vi "Simulation Resource Buffer.vi"(6 "IO Buffer Operation":T1, 8 "error in (no error)":errorcluster, 11 "Data in":variant) -> (0 "error out":errorcluster, 2 "Timed Out?":bool, 3 "Data out":variant)   [LabVIEW 2016]
uses:
  Typedefs/IO Buffer Operation.ctl
  Typedefs/IO Data Cluster.ctl
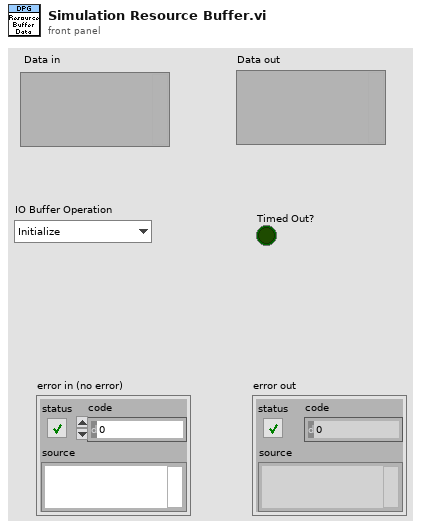
[diagram p1: front panel]
types:
  T1 = typedef "IO Buffer Operation.ctl" = enum16{"Initialize", "Write IO Data_Rd", "Read IO Data_Rd", "Write IO Data_Wr", "Read IO Data_Wr", "Write  IO Data_Dir", "Read  IO Data_Dir", "Write Host to Target FIFO", "Read Host to Target FIFO", "Write Target to Host FIFO", "Read Target to Host FIFO", "Write Monitor Enable?", "Read Monitor Enable?", "Close"}
  T2 = typedef "IO Data Cluster.ctl" = cluster{"Host to Target FIFO":refnum<queue>, "Target to Host FIFO":refnum<queue>, "Monitor Enable?":bool, "IO Data_Wr":refnum<queue>, "IO Data_Rd":refnum<queue>, "IO Data_Dir":u32}
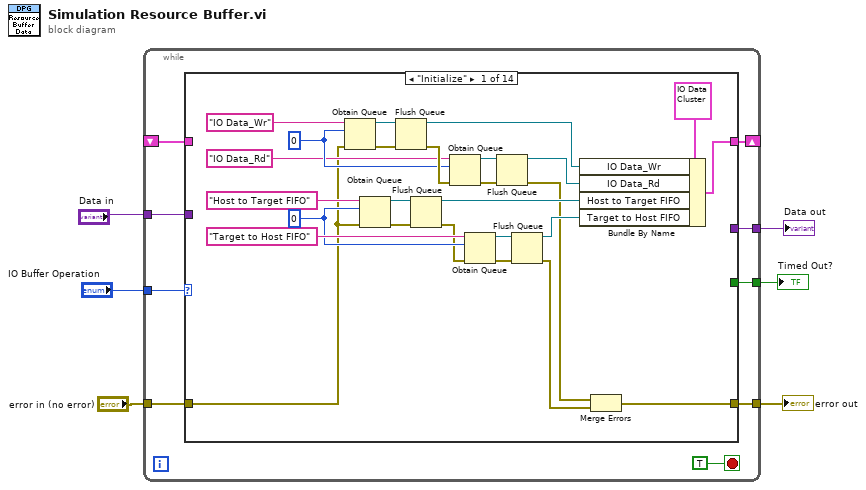
[diagram p0: block diagram]
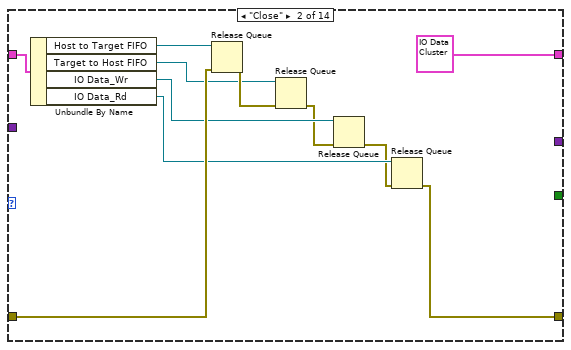
[diagram p2: hidden frame]
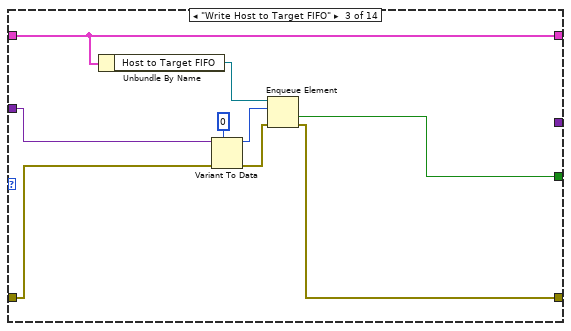
[diagram p3: hidden frame]
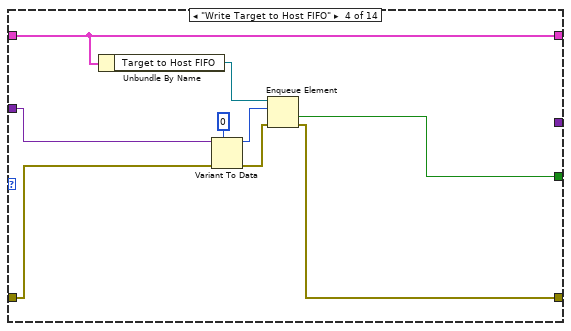
[diagram p4: hidden frame]
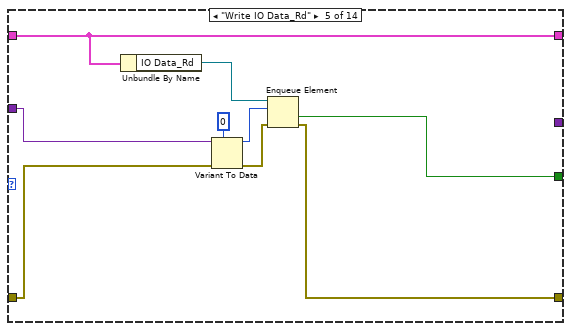
[diagram p5: hidden frame]
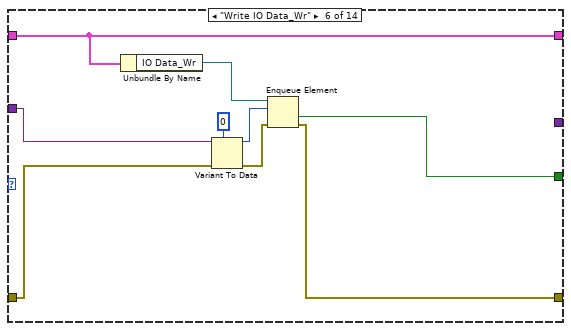
[diagram p6: hidden frame]
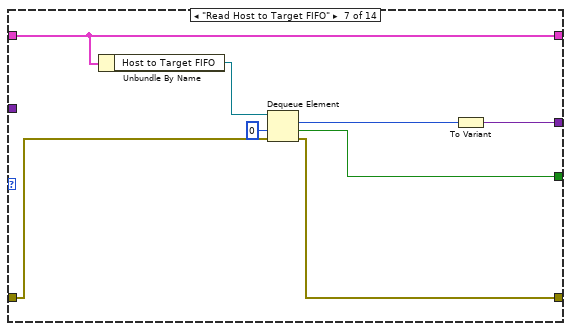
[diagram p7: hidden frame]
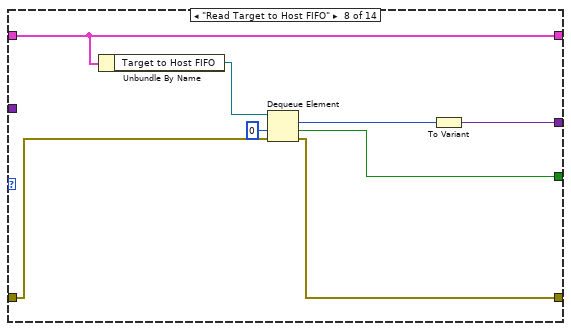
[diagram p8: hidden frame]
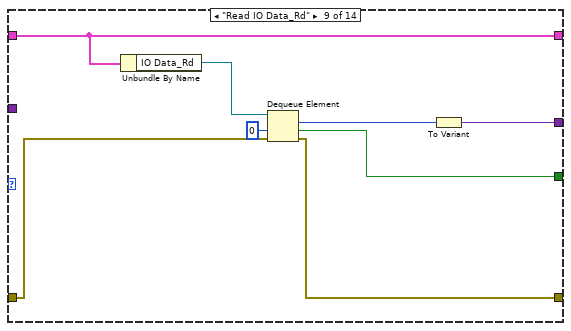
[diagram p9: hidden frame]
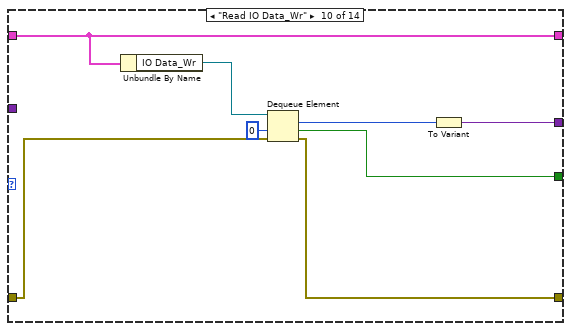
[diagram p10: hidden frame]
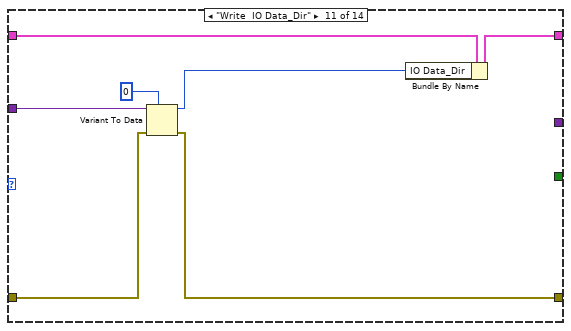
[diagram p11: hidden frame]
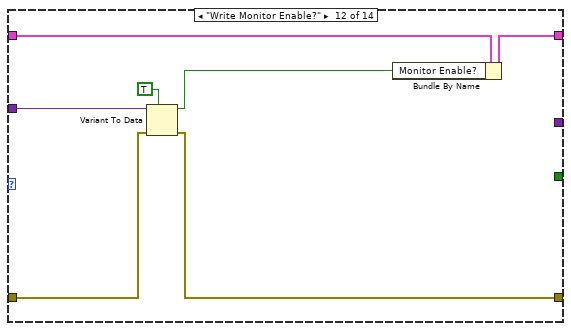
[diagram p12: hidden frame]
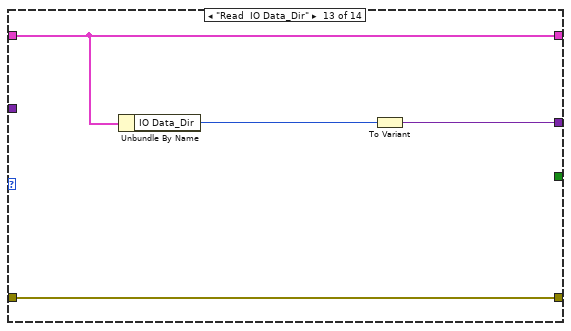
[diagram p13: hidden frame]
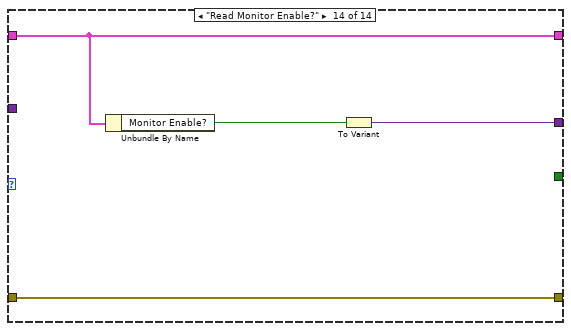
[diagram p14: hidden frame]
diagram:
  n1 = while {
    tunnel: "IO Buffer Operation" -> [w14]
    tunnel: "error in (no error)" -> [w9]
    tunnel: [w8] -> w5
    tunnel: "Data in" -> [w11]
    shift-right: [w13] -> _
    shift-left: _ -> [w12]
    tunnel: [w10] -> w2
    tunnel: [w7] -> w1
    stop <- TRUE stop-if-true
    n2 = case shown="\"Initialize\"" w14 {
      tunnel: [w37 T2 {"Host to Target FIFO"=refnum, "Target to Host FIFO"=refnum, "Monitor Enable?"=FALSE, "IO Data_Wr"=refnum, "IO Data_Rd"=refnum, "IO Data_Dir"=0} ("IO Data Cluster") w61 w70 w79 w88 w96 w104 w112 w120 w127 w134 w138 w142] -> w13
      tunnel: w12 -> [_ w50 w61 w70 w79 w88 w96 w104 w112 w120 w126 w133 w138 w142]
      tunnel: w11 -> [_ _ w59 w68 w77 w86 _ _ _ _ w123 w131 _ _]
      tunnel: [_ _ _ _ _ _ w90 w98 w106 w114 _ _ w135 w139] -> w10
      tunnel: [w17 w42 w54 w63 w72 w81 w94 w102 w110 w118 w122 w130 w136 w141] -> w8
      tunnel: w9 -> [w20 w51 w56 w65 w74 w83 w93 w101 w109 w117 w124 w132 w136 w141]
      tunnel: [_ _ w53 w62 w71 w80 w89 w97 w105 w113 _ _ _ _] -> w7
      frame "Initialize" {
        w23 = u32 0 ("Numeric")
        w39 = u64 0 ("Numeric")
        n3 = Obtain Queue(name (unnamed)="IO Data_Wr", element data type=w23, error in (no error)=w20) -> (queue out=w24:refnum<queue>, error out=w27:errorcluster)  [unwired: 2 in, 1 out]
        n4 = Obtain Queue(name (unnamed)="Host to Target FIFO", element data type=w39, error in (no error)=w20) -> (queue out=w36:refnum<queue>, error out=w31:errorcluster)  [unwired: 2 in, 1 out]
        n5 = Flush Queue(queue=w24, error in (no error)=w27) -> (queue out=w19:refnum<queue>, error out=w28:errorcluster)  [unwired: 1 out]
        n6 = Flush Queue(queue=w36, error in (no error)=w31) -> (queue out=w32:refnum<queue>, error out=w29:errorcluster)  [unwired: 1 out]
        n7 = Obtain Queue(name (unnamed)="IO Data_Rd", element data type=w23, error in (no error)=w28) -> (queue out=w25:refnum<queue>, error out=w26:errorcluster)  [unwired: 2 in, 1 out]
        n8 = Obtain Queue(name (unnamed)="Target to Host FIFO", element data type=w39, error in (no error)=w29) -> (queue out=w35:refnum<queue>, error out=w33:errorcluster)  [unwired: 2 in, 1 out]
        n9 = Flush Queue(queue=w25, error in (no error)=w26) -> (queue out=w18:refnum<queue>, error out=w16:errorcluster)  [unwired: 1 out]
        n10 = Flush Queue(queue=w35, error in (no error)=w33) -> (queue out=w34:refnum<queue>, error out=w30:errorcluster)  [unwired: 1 out]
        n11 = Bundle By Name(cluster=T2 {"Host to Target FIFO"=refnum, "Target to Host FIFO"=refnum, "Monitor Enable?"=FALSE, "IO Data_Wr"=refnum, "IO Data_Rd"=refnum, "IO Data_Dir"=0} ("IO Data Cluster"), "IO Data_Wr"=w19, "IO Data_Rd"=w18, "Host to Target FIFO"=w32, "Target to Host FIFO"=w34) -> (w37:T2)
        n12 = Merge Errors(w16, w30) -> (w17:errorcluster)
      }
      frame "Close" {
        n13 = Unbundle By Name(w50) -> ("Host to Target FIFO"=w49:refnum<queue>, "Target to Host FIFO"=w48:refnum<queue>, "IO Data_Wr"=w46:refnum<queue>, "IO Data_Rd"=w45:refnum<queue>)
        n14 = Release Queue(queue=w49, error in (no error)=w51) -> (error out=w52:errorcluster)  [unwired: 1 in, 2 out]
        n15 = Release Queue(queue=w48, error in (no error)=w52) -> (error out=w44:errorcluster)  [unwired: 1 in, 2 out]
        n16 = Release Queue(queue=w46, error in (no error)=w44) -> (error out=w43:errorcluster)  [unwired: 1 in, 2 out]
        n17 = Release Queue(queue=w45, error in (no error)=w43) -> (error out=w42:errorcluster)  [unwired: 1 in, 2 out]
      }
      frame "Write Host to Target FIFO" {
        n18 = Unbundle By Name(w61) -> ("Host to Target FIFO"=w60:refnum<queue>)
        n19 = Variant To Data(error in=w56, type=u64 0, Variant=w59) -> (data=w58:u64, error out=w55:errorcluster)
        n20 = Enqueue Element(queue=w60, element=w58, error in (no error)=w55) -> (timed out?=w53:bool, error out=w54:errorcluster)  [unwired: 1 in, 1 out]
      }
      frame "Write Target to Host FIFO" {
        n21 = Unbundle By Name(w70) -> ("Target to Host FIFO"=w69:refnum<queue>)
        n22 = Variant To Data(error in=w65, type=u64 0, Variant=w68) -> (data=w67:u64, error out=w64:errorcluster)
        n23 = Enqueue Element(queue=w69, element=w67, error in (no error)=w64) -> (timed out?=w62:bool, error out=w63:errorcluster)  [unwired: 1 in, 1 out]
      }
      frame "Write IO Data_Rd" {
        n24 = Unbundle By Name(w79) -> ("IO Data_Rd"=w78:refnum<queue>)
        n25 = Variant To Data(error in=w74, type=u32 0, Variant=w77) -> (data=w76:u32, error out=w73:errorcluster)
        n26 = Enqueue Element(queue=w78, element=w76, error in (no error)=w73) -> (timed out?=w71:bool, error out=w72:errorcluster)  [unwired: 1 in, 1 out]
      }
      frame "Write IO Data_Wr" {
        n27 = Unbundle By Name(w88) -> ("IO Data_Wr"=w87:refnum<queue>)
        n28 = Variant To Data(error in=w83, type=u32 0, Variant=w86) -> (data=w85:u32, error out=w82:errorcluster)
        n29 = Enqueue Element(queue=w87, element=w85, error in (no error)=w82) -> (timed out?=w80:bool, error out=w81:errorcluster)  [unwired: 1 in, 1 out]
      }
      frame "Read Host to Target FIFO" {
        n30 = Unbundle By Name(w96) -> ("Host to Target FIFO"=w95:refnum<queue>)
        n31 = Dequeue Element(queue=w95, timeout in ms (-1)=0, error in (no error)=w93) -> (element=w91:u64, timed out?=w89:bool, error out=w94:errorcluster)  [unwired: 1 out]
        n32 = To Variant(anything=w91) -> (Variant=w90:variant)
      }
      frame "Read Target to Host FIFO" {
        n33 = Unbundle By Name(w104) -> ("Target to Host FIFO"=w103:refnum<queue>)
        n34 = Dequeue Element(queue=w103, timeout in ms (-1)=0, error in (no error)=w101) -> (element=w100:u64, timed out?=w97:bool, error out=w102:errorcluster)  [unwired: 1 out]
        n35 = To Variant(anything=w100) -> (Variant=w98:variant)
      }
      frame "Read IO Data_Rd" {
        n36 = Unbundle By Name(w112) -> ("IO Data_Rd"=w111:refnum<queue>)
        n37 = Dequeue Element(queue=w111, timeout in ms (-1)=0, error in (no error)=w109) -> (element=w108:u32, timed out?=w105:bool, error out=w110:errorcluster)  [unwired: 1 out]
        n38 = To Variant(anything=w108) -> (Variant=w106:variant)
      }
      frame "Read IO Data_Wr" {
        n39 = Unbundle By Name(w120) -> ("IO Data_Wr"=w119:refnum<queue>)
        n40 = Dequeue Element(queue=w119, timeout in ms (-1)=0, error in (no error)=w117) -> (element=w116:u32, timed out?=w113:bool, error out=w118:errorcluster)  [unwired: 1 out]
        n41 = To Variant(anything=w116) -> (Variant=w114:variant)
      }
      frame "Write  IO Data_Dir" {
        n42 = Variant To Data(error in=w124, type=u32 0, Variant=w123) -> (data=w121:u32, error out=w122:errorcluster)
        n43 = Bundle By Name(cluster=w126, "IO Data_Dir"=w121) -> (w127:T2)
      }
      frame "Write Monitor Enable?" {
        n44 = Variant To Data(error in=w132, type=TRUE, Variant=w131) -> (data=w129:bool, error out=w130:errorcluster)
        n45 = Bundle By Name(cluster=w133, "Monitor Enable?"=w129) -> (w134:T2)
      }
      frame "Read  IO Data_Dir" {
        n46 = Unbundle By Name(w138) -> ("IO Data_Dir"=w137:u32)
        n47 = To Variant(anything=w137) -> (Variant=w135:variant)
      }
      frame "Read Monitor Enable?" {
        n48 = Unbundle By Name(w142) -> ("Monitor Enable?"=w140:bool)
        n49 = To Variant(anything=w140) -> (Variant=w139:variant)
      }
    }
  }
  "error out" <- w5
  "Data out" <- w2
  "Timed Out?" <- w1
